vi "buildSecondDatafromHalfHourData.vi"(2 "2015 data.csv":path, 3 "offsetHour":i32) -> (1 "Array":dbl[][](array[numeric]))   [LabVIEW 2013]
doc: "this subVI uses the \"2015 data.csv\" file. The current half hour information is parsed into a new array so that the information appears to change each second, rather than each half hour.\nThe day is always 30APR2015; utlize the hourOffset variable if you'd like to move the time away from your current system clock time."
uses:
  <vilib>/Utility/file.llb/Read From Spreadsheet File (DBL).vi
panel:
  out "nextRow":i32
  out "curRow":i32
  out "element":dbl format="%0.8f"
  out "rowCountOffset":i32
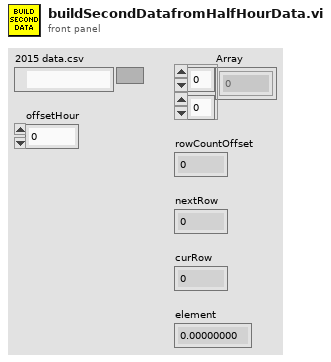
[diagram p1: front panel]
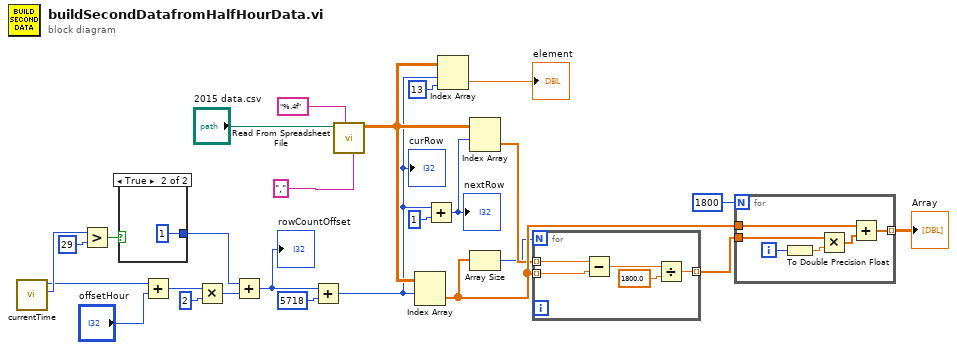
[diagram p0: block diagram]
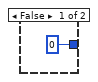
[diagram p2: hidden frame]
diagram:
  n1 = call "currentTime.vi"() -> ("Hour"=w4:i32, "Minute"=w6:i32)  [unwired: 6 in, 1 out]
  n2 = Greater?(x=w6, y=29) -> (0:w5:bool)
  n3 = case shown="True" w5 {
    tunnel: [0 ("y") 1 ("y")] -> w8
    frame False {
    }
    frame True {
    }
  }
  n4 = Add(x=w4, y="offsetHour") -> (x+y=w3:i32)
  n5 = Multiply(x=w3, y=2) -> (x*y=w9:i32)
  n6 = Add(x=w8, y=w9) -> (x+y=w16:i32)
  "rowCountOffset" <- w16
  n7 = Add(x=w16, y=5718 ("index (row)")) -> (x+y=w18:i32)
  "curRow" <- w18
  n8 = call-poly <vilib>:"Read From Spreadsheet File.vi"("delimiter (\\t)"="," ("delimiter (\\t)"), "format (%.3f)"="%.4f" ("format (%d)"), "file path (dialog if empty)"="2015 data.csv") -> ("all rows"=w20:dbl[][])  [unwired: 4 in, 4 out]
  n9 = Index Array(array=w20, index (row)=w18) -> (element=w24:dbl[])  [unwired: 1 in]
  n10 = Add(x=w18, y=1 ("index (row)")) -> (x+y=w19:i32)
  "nextRow" <- w19
  n11 = Index Array(array=w20, index (row)=w18, index (col)=13 ("disabled index (col)")) -> (element=→"element":dbl)
  n12 = Index Array(array=w20, index (row)=w19) -> (element=w22:dbl[])  [unwired: 1 in]
  n13 = Array Size(array=w24) -> (size(s)=w21:i32)
  n14 = for {
    N: w21 -> [_]
    tunnel: w24 -> [w32] mode=indexing
    tunnel: w22 -> [w33] mode=indexing
    tunnel: [w29] -> w25 mode=indexing
    n15 = Subtract(x=w33, y=w32) -> (x-y=w31:dbl)
    n16 = Divide(x=w31, y=1800.0 ("index (row)")) -> (x/y=w29:dbl)
  }
  n17 = for {
    N: 1800 ("index (row)") -> [_]
    tunnel: w24 -> [w35]
    tunnel: w25 -> [w37]
    tunnel: [w34] -> w26 mode=indexing
    i -> [w39]
    n18 = To Double Precision Float(number=w39) -> (double precision float=w38:dbl)
    n19 = Multiply(x=w37, y=w38) -> (x*y=w36:dbl[])
    n20 = Add(x=w35, y=w36) -> (x+y=w34:dbl[])
  }
  "Array" <- w26
